vi "6060_set_all_outputs.vi"(1 "Address (Main only)":T1, 2 "Digital output state byte":u16 max=63 format="%.0b") -> (3 "Comment":string, 6 "Good Reply":bool)   [LabVIEW 2020]
uses:
  ADAM Client/Sub VIs/ADAM Controls/Address.ctl
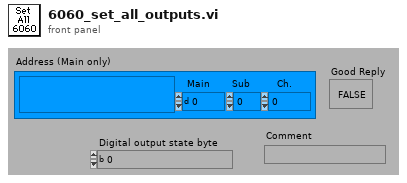
[diagram p1: front panel]
types:
  T1 = typedef "Address.ctl" = cluster{"Main":i32, "Ch.":i32, "Sub":i32, "Port Name":string}
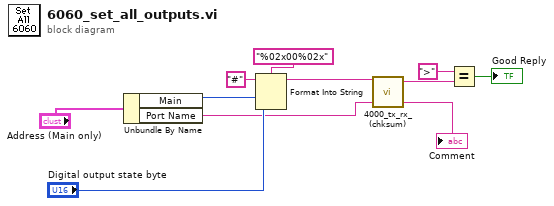
[diagram p0: block diagram]
diagram:
  n1 = Unbundle By Name("Address (Main only)") -> ("Main"=w11:i32, "Port Name"=w4:string)
  n2 = Format Into String(format string="%02x00%02x", initial string="#", w11, "Digital output state byte") -> (resulting string=w8:string)  [unwired: 1 in, 1 out]
  n3 = call "4000_tx_rx_(chksum).vi"("Write String"=w8, "Port Name"=w4) -> ("Read"=w1:string, "Comment out"=→"Comment":string)  [unwired: 3 in, 1 out]
  n4 = Equal?(x=">", y=w1) -> (x = y?=→"Good Reply":bool)
